vi "Configure Protection.vi"(6 "Protection (None)":T1, 8 "error in":errorcluster, 10 "Limit":dbl, 11 "6700 in":refnum<class "6700.lvclass">) -> (0 "error out":errorcluster, 3 "6700 out":refnum<class "6700.lvclass">)   [LabVIEW 2018, in "6700.lvlib" / "6700.lvclass"]
doc: "Configure Protection setting, available options:\n\n0: None\n1: Over Voltage\n2: Under Voltage\n3: Over Current\n\nDbl Precision Limit"
uses:
  6700.lvclass
  builds/Power_Supply.lvlibp/Custom Control/Protection.ctl
  6700.lvclass/6700.ctl
  <instrlib>/Agilent N6700 Series/Agilent N6700 Series.lvlib
  builds/Power_Supply.lvlibp/Power Supply.lvclass
  C:/Users/Ron.Dexter.LUMINARTECH/Desktop/builds/Power_Supply.lvlibp/Power Supply.lvclass
  builds/Power_Supply.lvlibp
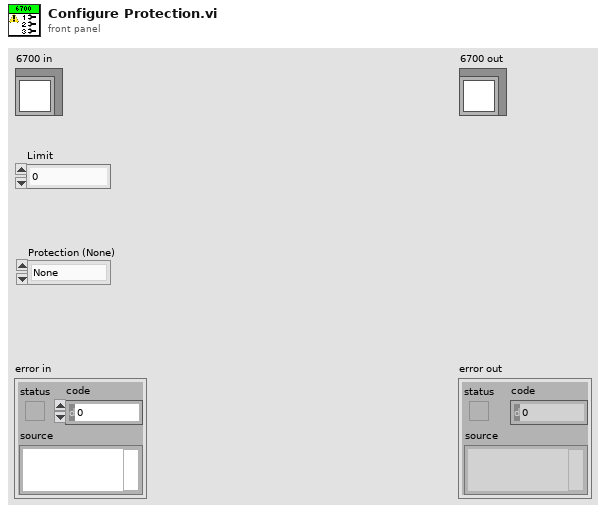
[diagram p1: front panel]
types:
  T1 = typedef "Power_Supply.lvlibp/Protection.ctl" = enum16{"None", "Over Volt", "Under Volt", "Over Current"}
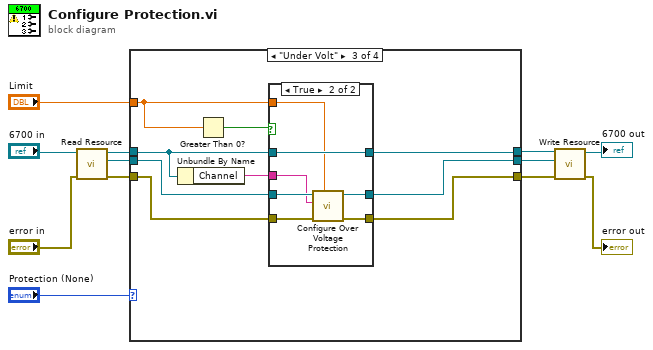
[diagram p0: block diagram]
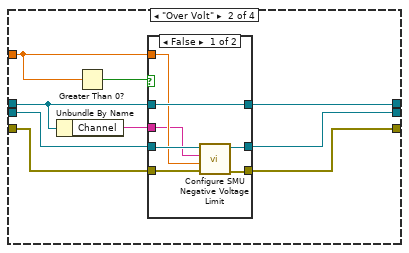
[diagram p3: hidden frame]
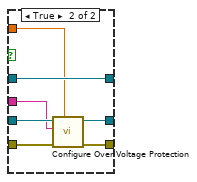
[diagram p4: hidden frame]
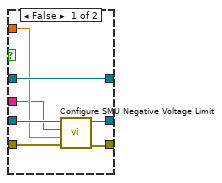
[diagram p5: hidden frame]
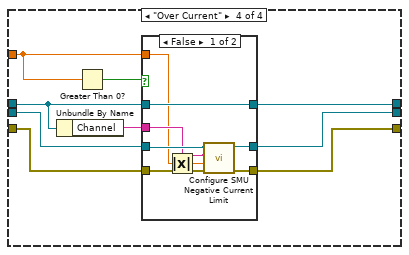
[diagram p6: hidden frame]
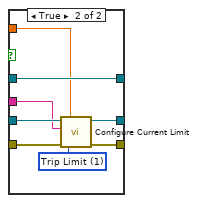
[diagram p7: hidden frame]
diagram:
  n1 = call "Read Resource.vi"("error in"="error in", "Power Supply in"="6700 in") -> ("error out"=w7:errorcluster, "Resource"=w8:refnum<visa-resource-name>, "Power Supply out"=w9:refnum<class "6700.lvclass">)  [unwired: 7 in]
  n2 = case shown="\"Under Volt\"" "Protection (None)" {
    tunnel: w9 -> [w15 w20 w43 w66]
    tunnel: "Limit" -> [_ w23 w46 w69]
    tunnel: [w15 w17 w40 w63] -> w4
    tunnel: w8 -> [w13 w22 w45 w68]
    tunnel: w7 -> [w14 w21 w44 w67]
    tunnel: [w13 w18 w41 w64] -> w5
    tunnel: [w14 w16 w39 w62] -> w3
    frame "None", Default {
    }
    frame "Over Volt" {
      n3 = Unbundle By Name(w20) -> ("Channel"=w19:string)
      n4 = Greater Than 0?(x=w23) -> (x > 0?=w24:bool)
      n5 = case shown="False" w24 {
        tunnel: w22 -> [w27 w38]
        tunnel: w21 -> [w30 w37]
        tunnel: [w29 w36] -> w16
        tunnel: [w28 w35] -> w18
        tunnel: w20 -> [w31 w34]
        tunnel: [w31 w34] -> w17
        tunnel: w23 -> [w26 w33]
        tunnel: w19 -> [w25 w32]
        frame False {
          n6 = call <instrlib>:"Configure SMU Negative Voltage Limit.vi"("error in (no error)"=w30, "Negative Voltage Limit (0.0 volts)"=w26, "Channel Name (1)"=w25, "VISA resource name"=w27) -> ("error out"=w29:errorcluster, "VISA resource name out"=w28:refnum<visa-resource-name>)  [unwired: 6 in]
        }
        frame True {
          n7 = call <instrlib>:"Configure Over Voltage Protection.vi"("Limit (0.0 volts)"=w33, "error in (no error)"=w37, "Channel Name (1)"=w32, "VISA resource name"=w38) -> ("error out"=w36:errorcluster, "VISA resource name out"=w35:refnum<visa-resource-name>)  [unwired: 6 in]
        }
      }
    }
    frame "Under Volt" {
      n8 = Unbundle By Name(w43) -> ("Channel"=w42:string)
      n9 = Greater Than 0?(x=w46) -> (x > 0?=w47:bool)
      n10 = case shown="True" w47 {
        tunnel: w45 -> [w50 w61]
        tunnel: w44 -> [w53 w60]
        tunnel: [w52 w59] -> w39
        tunnel: [w51 w58] -> w41
        tunnel: w43 -> [w54 w57]
        tunnel: [w54 w57] -> w40
        tunnel: w46 -> [w49 w56]
        tunnel: w42 -> [w48 w55]
        frame False {
          n11 = call <instrlib>:"Configure SMU Negative Voltage Limit.vi"("error in (no error)"=w53, "Negative Voltage Limit (0.0 volts)"=w49, "Channel Name (1)"=w48, "VISA resource name"=w50) -> ("error out"=w52:errorcluster, "VISA resource name out"=w51:refnum<visa-resource-name>)  [unwired: 6 in]
        }
        frame True {
          n12 = call <instrlib>:"Configure Over Voltage Protection.vi"("Limit (0.0 volts)"=w56, "error in (no error)"=w60, "Channel Name (1)"=w55, "VISA resource name"=w61) -> ("error out"=w59:errorcluster, "VISA resource name out"=w58:refnum<visa-resource-name>)  [unwired: 6 in]
        }
      }
    }
    frame "Over Current" {
      n13 = Unbundle By Name(w66) -> ("Channel"=w65:string)
      n14 = Greater Than 0?(x=w69) -> (x > 0?=w70:bool)
      n15 = case shown="False" w70 {
        tunnel: w68 -> [w74 w82]
        tunnel: w67 -> [w77 w85]
        tunnel: [w76 w84] -> w62
        tunnel: [w75 w83] -> w64
        tunnel: w66 -> [w78 w86]
        tunnel: [w78 w86] -> w63
        tunnel: w69 -> [w71 w81]
        tunnel: w65 -> [w73 w80]
        frame False {
          n16 = Absolute Value(x=w71) -> (abs(x)=w72:dbl)
          n17 = call <instrlib>:"Configure SMU Negative Current Limit.vi"("error in (no error)"=w77, "Negative Current Limit (0.0 amps)"=w72, "Channel Name (1)"=w73, "VISA resource name"=w74) -> ("error out"=w76:errorcluster, "VISA resource name out"=w75:refnum<visa-resource-name>)  [unwired: 6 in]
        }
        frame True {
          w79 = 1 items=["Regulatory Limit", "Trip Limit"] ("Behavior (0: Regulatory Limit)")
          n18 = call <instrlib>:"Configure Current Limit.vi"("Limit (0.0 amps)"=w81, "error in (no error)"=w85, "Behavior (0: Regulatory Limit)"=w79, "Channel Name (1)"=w80, "VISA resource name"=w82) -> ("error out"=w84:errorcluster, "VISA resource name out"=w83:refnum<visa-resource-name>)  [unwired: 5 in]
        }
      }
    }
  }
  n19 = call "Write Resource.vi"("error in"=w3, "Resource"=w5, "Power Supply in"=w4) -> ("error out"=→"error out":errorcluster, "Power Supply out"=→"6700 out":refnum<class "6700.lvclass">)  [unwired: 7 in]
